vi "Print Console.vi"() -> ()   [LabVIEW 2018]
doc: "인쇄 작업 제출을 컨트롤하고 인쇄 작업의 처리 상태를 모니터"
panel:
  out "인쇄 LED":cluster{"대기 중":bool, "초기화 중":bool, "인쇄 중":bool}={"대기 중"=TRUE, "초기화 중"=FALSE, "인쇄 중"=FALSE}
  in  "정지 버튼":bool
  in  "큐 이벤트":bool
  out "큐 인쇄 작업":i32(slide) scale=0.0..25.0
  # "큐 인쇄 작업"
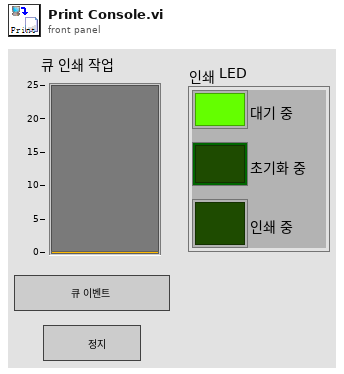
[diagram p1: front panel]
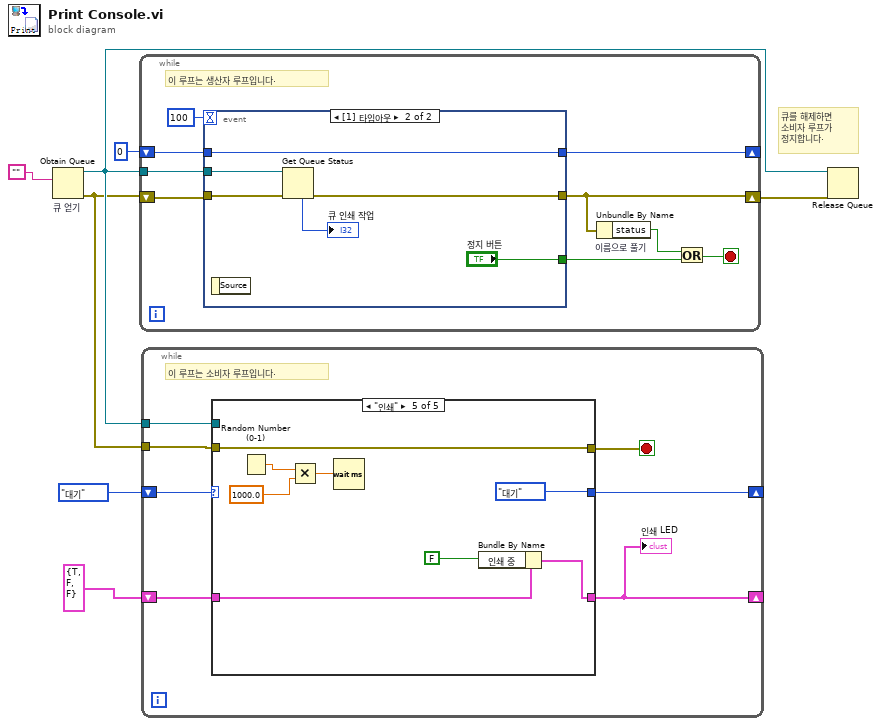
[diagram p0: block diagram]
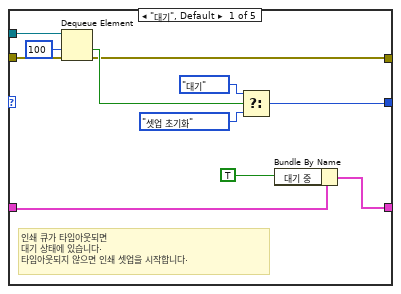
[diagram p2: hidden frame]
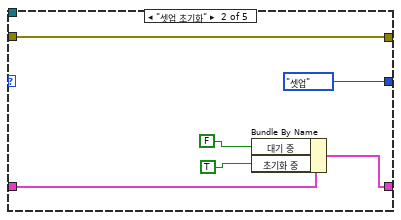
[diagram p3: hidden frame]
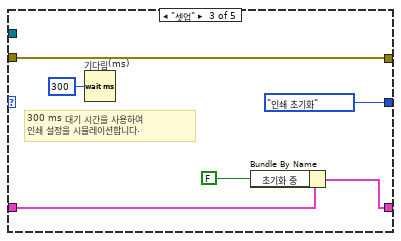
[diagram p4: hidden frame]
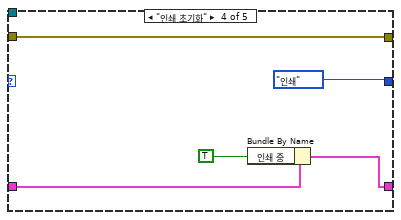
[diagram p5: hidden frame]
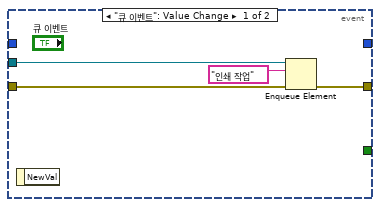
[diagram p6: hidden frame]
diagram:
  # "큐를 해제하면\n소비자 루프가\n정지합니다."
  n1 = Obtain Queue "큐 얻기"(element data type="") -> (queue out=w5:refnum<queue>, error out=w1:errorcluster)  [unwired: 4 in, 1 out]
  n2 = while {
    tunnel: w5 -> [w15]
    shift-right: [w12] -> w7
    shift-left: w1 -> [w14]
    shift-right: [w8] -> _
    shift-left: 0 -> [w9]
    stop <- w13 stop-if-true
    # "이 루프는 생산자 루프입니다."
    n3 = event shown="[1] 타임아웃" {
      selector: _ -> [_ _]
      dyn-events: _ -> [_ _]
      timeout: 100 -> [_ _]
      tunnel: w15 -> [w19 w26]
      tunnel: w14 -> [w18 w25]
      tunnel: [w17 w24] -> w12
      tunnel: [_ "정지 버튼"] -> w10
      tunnel: [_ w22] -> w8
      tunnel: w9 -> [_ w22]
      event "큐 이벤트": Value Change {
        n4 = event-data() -> ()  [unwired: 1 in, 1 out]
        n5 = Enqueue Element(queue=w19, element="인쇄 작업" ("원소"), error in (no error)=w18) -> (error out=w17:errorcluster)  [unwired: 1 in, 2 out]
      }
      event Timeout {
        n6 = event-data() -> ()  [unwired: 1 in, 1 out]
        n7 = Get Queue Status(queue=w26, error in (no error)=w25) -> (error out=w24:errorcluster, # elements in queue=→"큐 인쇄 작업":i32)  [unwired: 1 in, 6 out]
      }
    }
    n8 = Unbundle By Name "이름으로 풀기"(w12) -> ("status"=w11:bool)
    n9 = Or(x=w11, y=w10) -> (x .or. y?=w13:bool)
  }
  n10 = while {
    shift-right: [w29] -> _
    shift-left: cluster{"대기 중":bool, "초기화 중":bool, "인쇄 중":bool} {"대기 중"=TRUE, "초기화 중"=FALSE, "인쇄 중"=FALSE} ("에러 상수") -> [w30]
    shift-right: [w31] -> _
    shift-left: enum16{"대기", "셋업 초기화", "셋업", "인쇄 초기화", "인쇄"}."대기" -> [w33]
    tunnel: w5 -> [w32]
    tunnel: w1 -> [w28]
    stop <- w27 stop-if-true
    # "이 루프는 소비자 루프입니다."
    n11 = case shown="\"인쇄\"" w33 {
      tunnel: w32 -> [w43 _ _ _ _]
      tunnel: [w42 enum16{"대기", "셋업 초기화", "셋업", "인쇄 초기화", "인쇄"}."셋업" enum16{"대기", "셋업 초기화", "셋업", "인쇄 초기화", "인쇄"}."인쇄 초기화" enum16{"대기", "셋업 초기화", "셋업", "인쇄 초기화", "인쇄"}."인쇄" enum16{"대기", "셋업 초기화", "셋업", "인쇄 초기화", "인쇄"}."대기"] -> w31
      tunnel: [w38 w46 w53 w59 w65] -> w29
      tunnel: w30 -> [w37 w49 w54 w60 w66]
      tunnel: w28 -> [w35 w45 w51 w57 w62]
      tunnel: [w34 w45 w51 w57 w62] -> w27
      frame "대기", Default {
        # "인쇄 큐가 타임아웃되면\n대기 상태에 있습니다.\n타임아웃되지 않으면 인쇄 셋업을 시작합니다."
        n12 = Dequeue Element(queue=w43, timeout in ms (-1)=100 ("타임아웃(ms) (-1)"), error in (no error)=w35) -> (timed out?=w41:bool, error out=w34:errorcluster)  [unwired: 2 out]
        n13 = Select(t=enum16{"대기", "셋업 초기화", "셋업", "인쇄 초기화", "인쇄"}."대기", s=w41, f=enum16{"대기", "셋업 초기화", "셋업", "인쇄 초기화", "인쇄"}."셋업 초기화") -> (s? t:f=w42:enum16{"대기", "셋업 초기화", "셋업", "인쇄 초기화", "인쇄"})
        n14 = Bundle By Name(cluster=w37, "대기 중"=TRUE) -> (w38:cluster{"대기 중":bool, "초기화 중":bool, "인쇄 중":bool})
      }
      frame "셋업 초기화" {
        n15 = Bundle By Name(cluster=w49, "대기 중"=FALSE, "초기화 중"=TRUE) -> (w46:cluster{"대기 중":bool, "초기화 중":bool, "인쇄 중":bool})
      }
      frame "셋업" {
        # "300 ms 대기 시간을 사용하여\n인쇄 설정을 시뮬레이션합니다."
        n16 = Wait (ms) "기다림(ms)"(milliseconds to wait=u32 300 ("대기 시간 (ms)")) -> ()  [unwired: 1 out]
        n17 = Bundle By Name(cluster=w54, "초기화 중"=FALSE) -> (w53:cluster{"대기 중":bool, "초기화 중":bool, "인쇄 중":bool})
      }
      frame "인쇄 초기화" {
        n18 = Bundle By Name(cluster=w60, "인쇄 중"=TRUE) -> (w59:cluster{"대기 중":bool, "초기화 중":bool, "인쇄 중":bool})
      }
      frame "인쇄" {
        n19 = Random Number (0-1)() -> (number: 0 to 1=w69:dbl)
        n20 = Multiply(x=w69, y=1000.0) -> (x*y=w67:dbl)
        n21 = Wait (ms)(milliseconds to wait=w67) -> ()  [unwired: 1 out]
        n22 = Bundle By Name(cluster=w66, "인쇄 중"=FALSE) -> (w65:cluster{"대기 중":bool, "초기화 중":bool, "인쇄 중":bool})
      }
    }
    "인쇄 LED" <- w29
  }
  n23 = Release Queue(queue=w5, error in (no error)=w7) -> ()  [unwired: 1 in, 3 out]
